vi "spi_init.vi"() -> ()   [LabVIEW 2026]
uses:
  <vilib>/MakerHub/LINX/Private/Type Defs/Peripherals/SPI/SPI Configuration.ctl
  <vilib>/MakerHub/LINX/Private/Type Defs/Peripherals/SPI/SPI Bit Order.ctl
  <vilib>/MakerHub/LINX/Private/Type Defs/Peripherals/SPI/SPI Mode.ctl
  <vilib>/MakerHub/LINX/Public/Peripherals/SPI/SPI CS Config.ctl
  <vilib>/MakerHub/LINX/Private/Type Defs/Peripherals/SPI/SPI CS Logic Level.ctl
  <vilib>/MakerHub/LINX/Public/Peripherals/SPI/SPI Write Read N Frames.vi
  <vilib>/MakerHub/LINX/Private/Local IO/LinxSpiWriteRead.vi
  <vilib>/MakerHub/LINX/Public/Utilities/Check Channel.vi
  <vilib>/MakerHub/LINX/Public/Utilities/Open Serial.vi
  <vilib>/MakerHub/LINX/Private/Utilties/Generate Error.vi
  <vilib>/MakerHub/LINX/LMH-LINX.lvlib
panel:
  out "Data":u8
  out "i + 1":u8
  out "Array 2":u8[](array[numeric])
  in  "Array":bool[][](array[boolean])
  in  "CS Configuration":T1={"CS Channel"=7, "CS Logic Level"=enum."Active High"}
  in  "Stop Button":bool
  in  "SPI Configuration":T3={"Clock Frequency"=1000000, "Bit Order"=enum."LSb First", "SPI Mode"=enum."Mode 0"}
  in  "Serial Port":refnum<visa-resource-name>="N/A"
  # "Specify Serial Port"
  # "MAX7219 Matrix requires Most Significant Bit (MSb)!"
  # "Specify CS Pin on Arduino"
  # "MAX7219 required Active Low Chip Select!"
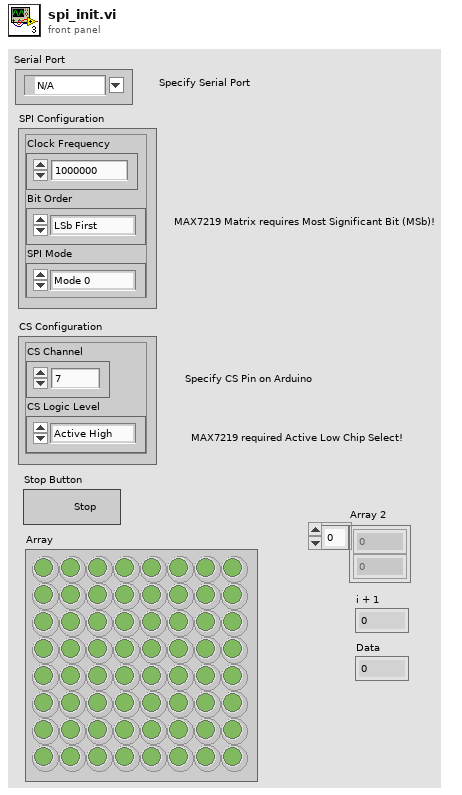
[diagram p1: front panel]
types:
  T1 = typedef "LMH-LINX.lvlib/SPI CS Config.ctl" = cluster{"CS Channel":u8, "CS Logic Level":T2}
  T2 = typedef "LMH-LINX.lvlib/SPI CS Logic Level.ctl" = enum8{"Active Low", "Active High"}
  T3 = typedef "LMH-LINX.lvlib/SPI Configuration.ctl" = cluster{"Clock Frequency":u32, "Bit Order":T4, "SPI Mode":T5}
  T4 = typedef "LMH-LINX.lvlib/SPI Bit Order.ctl" = enum8{"LSb First", "MSb First"}
  T5 = typedef "LMH-LINX.lvlib/SPI Mode.ctl" = enum8{"Mode 0", "Mode 1", "Mode 2", "Mode 3"}
  T6 = typedef "LMH-LINX.lvlib/LINX Ref.ctl" = cluster{"IO":T7, "Interface":T8, "LINX Device Config":T9}
  T7 = typedef "LMH-LINX.lvlib/Platform.ctl" = enum16{"Remote", "Local"}
  T8 = typedef "LMH-LINX.lvlib/Interface.ctl" = enum16{"Serial", "TCP"}
  T9 = typedef "LMH-LINX.lvlib/Device.lvlib/LINX Device Config.ctl" = cluster{"Interface":T8, "COM Port":refnum<visa-resource-name>, "TCP Configuration":T10, "Device Family":u8, "Device ID":u8, "Device Name":string, "TCP Ref":refnum<k5>, "Channels":T11}
  T10 = typedef "LMH-LINX.lvlib/Device.lvlib/TCP Config.ctl" = cluster{"IP Address":string, "Port":u16}
  T11 = typedef "LMH-LINX.lvlib/Channels.ctl" = cluster{"DI":u8[], "DO":u8[], "AI":u8[], "AO":u8[], "PWM":u8[], "QE":u8[], "UART":u8[], "I2C 2":u8[], "SPI":u8[], "CAN":u8[], "Servo":u8[], "AI Ref (V)":dbl, "AI Resolution (Bits)":u8, "AO Ref (V)":dbl, "AO Resolution (Bits)":u8}
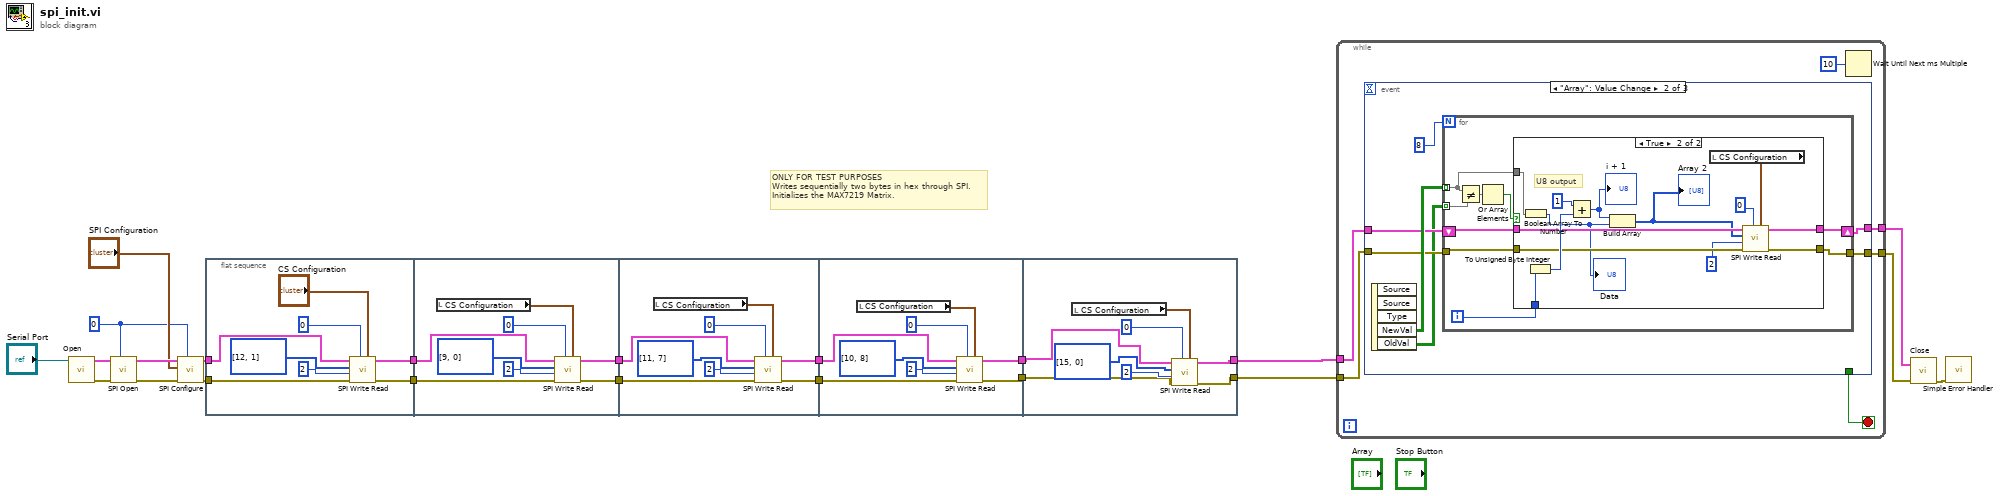
[diagram p0: block diagram]
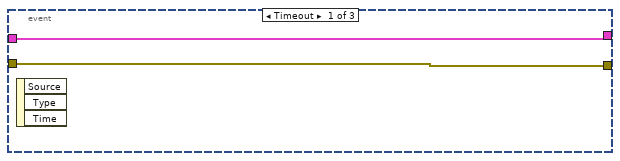
[diagram p2: hidden frame]
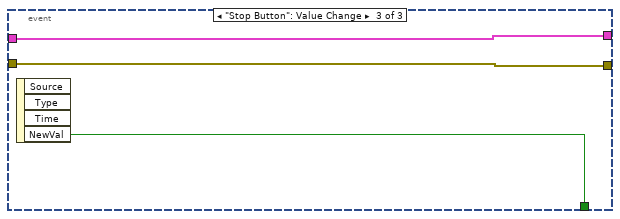
[diagram p4: hidden frame]
diagram:
  w15 = u8 0 ("SPI Channel (0)")
  # "ONLY FOR TEST PURPOSES\nWrites sequentially two bytes in hex through SPI.\nInitializes the MAX7219 Matrix."
  n1 = call-poly <vilib>:"Open.vi"("Serial Port"="Serial Port") -> ("Error Out"=w19:errorcluster, "LINX Resource"=w20:T6)  [unwired: 8 in, 1 out]
  n2 = call <vilib>:"SPI Open.vi"("SPI Channel (0)"=w15, "Error In"=w19, "LINX Resource"=w20) -> ("Error Out"=w17:errorcluster, "LINX Resource"=w18:T6)  [unwired: 7 in]
  n3 = call <vilib>:"SPI Configure.vi"("SPI Channel (0)"=w15, "Error In"=w17, "SPI Configuration"="SPI Configuration", "LINX Resource"=w18) -> ("Error Out"=w6:errorcluster, "LINX Resource"=w5:T6)  [unwired: 5 in, 1 out]
  n4 = flat-sequence {
    tunnel: [w28] -> w14
    tunnel: [w27] -> w13
    tunnel: w6 -> [w24]
    tunnel: w5 -> [w23]
    tunnel: w14 -> [w35]
    tunnel: w13 -> [w33]
    tunnel: [w34] -> w12
    tunnel: [w32] -> w11
    tunnel: w12 -> [w43]
    tunnel: [w42] -> w10
    tunnel: w11 -> [w41]
    tunnel: [w40] -> w9
    tunnel: w10 -> [w51]
    tunnel: w9 -> [w50]
    tunnel: [w48] -> w2
    tunnel: [w47] -> w1
    tunnel: [w57] -> w7
    tunnel: [w55] -> w8
    tunnel: w2 -> [w56]
    tunnel: w1 -> [w58]
    frame #0 {
      n5 = call-poly <vilib>:"SPI Write Read.vi"("CS Configuration"="CS Configuration", "SPI Channel (0)"=u8 0, "Error In"=w24, "SPI Frame Size"=u8 2, "Data"=u8[] [12, 1], "LINX Resource"=w23) -> ("Error Out"=w27:errorcluster, "LINX Resource"=w28:T6)  [unwired: 2 in, 2 out]
    }
    frame #1 {
      n6 = local read "CS Configuration"() -> (w31:T1)
      n7 = call-poly <vilib>:"SPI Write Read.vi"("CS Configuration"=w31, "SPI Channel (0)"=u8 0, "Error In"=w33, "SPI Frame Size"=u8 2, "Data"=u8[] [9, 0], "LINX Resource"=w35) -> ("Error Out"=w32:errorcluster, "LINX Resource"=w34:T6)  [unwired: 2 in, 2 out]
    }
    frame #2 {
      n8 = local read "CS Configuration"() -> (w39:T1)
      n9 = call-poly <vilib>:"SPI Write Read.vi"("CS Configuration"=w39, "SPI Channel (0)"=u8 0, "Error In"=w41, "SPI Frame Size"=u8 2, "Data"=u8[] [11, 7], "LINX Resource"=w43) -> ("Error Out"=w40:errorcluster, "LINX Resource"=w42:T6)  [unwired: 2 in, 2 out]
    }
    frame #3 {
      n10 = local read "CS Configuration"() -> (w49:T1)
      n11 = call-poly <vilib>:"SPI Write Read.vi"("CS Configuration"=w49, "SPI Channel (0)"=u8 0, "Error In"=w50, "SPI Frame Size"=u8 2, "Data"=u8[] [10, 8], "LINX Resource"=w51) -> ("Error Out"=w47:errorcluster, "LINX Resource"=w48:T6)  [unwired: 2 in, 2 out]
    }
    frame #4 {
      n12 = local read "CS Configuration"() -> (w62:T1)
      n13 = call-poly <vilib>:"SPI Write Read.vi"("CS Configuration"=w62, "SPI Channel (0)"=u8 0, "Error In"=w58, "SPI Frame Size"=u8 2, "Data"=u8[] [15, 0], "LINX Resource"=w56) -> ("Error Out"=w57:errorcluster, "LINX Resource"=w55:T6)  [unwired: 2 in, 2 out]
    }
  }
  n14 = while {
    tunnel: w7 -> [w65]
    tunnel: w8 -> [w67]
    tunnel: [w66] -> w4
    tunnel: [w64] -> w3
    stop <- w63 stop-if-true
    n15 = event shown="[1] \"Array\": Value Change" {
      selector: _ -> [_ _ _]
      dyn-events: _ -> [_ _ _]
      timeout: _ -> [_ _ _]
      tunnel: w67 -> [w70 w76 w105]
      tunnel: [w70 w75 w105] -> w66
      tunnel: w65 -> [w69 w74 w104]
      tunnel: [w69 w73 w104] -> w64
      tunnel: [_ _ w103] -> w63
      event Timeout {
        n16 = event-data() -> ()  [unwired: 1 in, 3 out]
      }
      event "Array": Value Change {
        n17 = event-data() -> ("NewVal"=w77:bool[][], "OldVal"=w71:bool[][])  [unwired: 1 in, 3 out]
        n18 = for {
          N: 8 -> [_]
          tunnel: w77 -> [w78] mode=indexing
          shift-right: [w83] -> w75
          shift-left: w76 -> [w85]
          tunnel: w74 -> [w84]
          tunnel: [w82] -> w73
          tunnel: w71 -> [w81] mode=indexing
          i -> [w86]
          n19 = Not Equal?(x=w78, y=w81) -> (x != y?=w80:bool[])
          n20 = Or Array Elements(Boolean array=w80) -> (logical OR=w79:bool)
          n21 = case shown="True" w79 {
            tunnel: w86 -> [_ w101]
            tunnel: w85 -> [w88 w97]
            tunnel: w84 -> [w87 w96]
            tunnel: [w88 w95] -> w83
            tunnel: [w87 w94] -> w82
            tunnel: w78 -> [_ w90]
            frame False {
            }
            frame True {
              # "U8 output"
              n22 = Boolean Array To Number(Boolean array=w90) -> (number=w91:u8)
              "Data" <- w91
              n23 = To Unsigned Byte Integer(number=w101) -> (unsigned 8bit integer=w100:u8)
              n24 = Add(x=u8 1 ("y"), y=w100) -> (x+y=w92:u8)
              "i + 1" <- w92
              n25 = Build Array(w92, w91) -> (w93:u8[])
              "Array 2" <- w93
              n26 = local read "CS Configuration"() -> (w98:T1)
              n27 = call-poly <vilib>:"SPI Write Read.vi"("CS Configuration"=w98, "SPI Channel (0)"=u8 0, "Error In"=w96, "SPI Frame Size"=u8 2, "Data"=w93, "LINX Resource"=w97) -> ("Error Out"=w94:errorcluster, "LINX Resource"=w95:T6)  [unwired: 2 in, 2 out]
            }
          }
        }
      }
      event "Stop Button": Value Change {
        n28 = event-data() -> ("NewVal"=w103:bool)  [unwired: 1 in, 3 out]
      }
    }
    n29 = Wait Until Next ms Multiple(millisecond multiple=u32 10) -> ()  [unwired: 1 out]
  }
  n30 = call <vilib>:"Close.vi"("Error In"=w3, "LINX Resource"=w4) -> ("Error Out"=w21:errorcluster)  [unwired: 9 in]
  n31 = call <vilib>:"Simple Error Handler.vi"("error in (no error)"=w21) -> ()  [unwired: 4 in, 5 out]
